vi "Post.vi"(8 "error in (no error)":errorcluster, 9 "PostRequest":string, 10 "Request":string, 11 "ByteGSWebAPI-V0 in":refnum<class "ByteGSWebAPI-V0.lvclass">) -> (0 "error out":errorcluster, 3 "ByteGSWebAPI-V0 out":refnum<class "ByteGSWebAPI-V0.lvclass">, 4 "body":string, 6 "headers":string)   [LabVIEW 2019, in "ByteGSWebAPI.lvlib" / "ByteGSWebAPI-V0.lvclass"]
uses:
  ByteGSWebAPI-V0.lvclass
  <vilib>/httpClient/POSTBuffer.vi
  <vilib>/httpClient/LabVIEWHTTPClient.lvlib
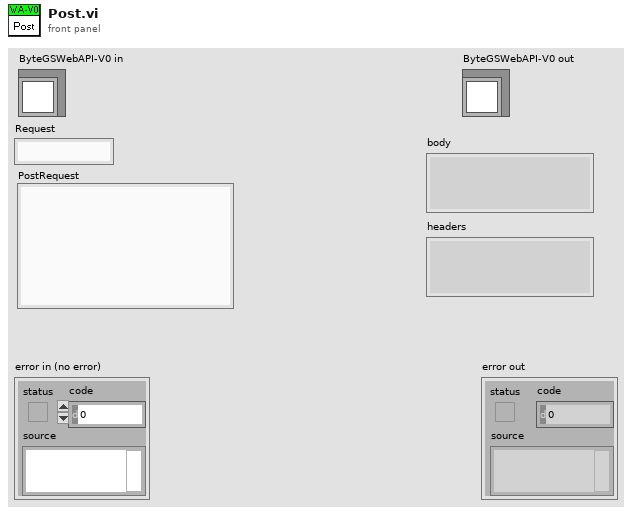
[diagram p1: front panel]
types:
  T1 = typedef "LabVIEWHTTPClient.lvlib/ClientHandle.ctl" = refnum<k1>
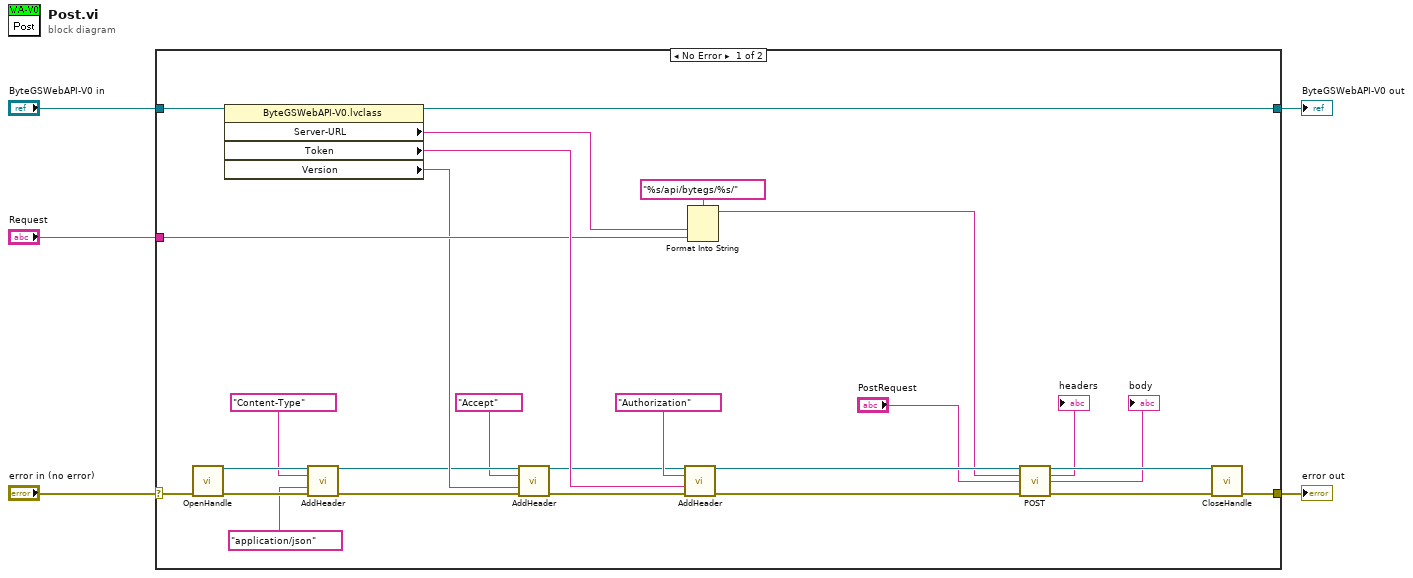
[diagram p0: block diagram]
diagram:
  n1 = case shown="No Error" "error in (no error)" {
    selector: "error in (no error)" -> [w27 w34]
    tunnel: [w26 w34] -> w4
    tunnel: [w25 w33] -> w2
    tunnel: "ByteGSWebAPI-V0 in" -> [w24 w33]
    tunnel: "Request" -> [w20 _]
    frame No Error {
      n2 = call <vilib>:"OpenHandle.vi"("error in (no error)"=w27) -> ("client handle out"=w30:T1, "error out"=w31:errorcluster)  [unwired: 13 in]
      n3 = property class="ByteGSWebAPI-V0.lvclass"(reference=w24) -> (reference out=w25:refnum<class "ByteGSWebAPI-V0.lvclass">, "Server-URL"=w21:string, "Token"=w23:string, "Version"=w19:string)  [unwired: 1 in, 1 out]
      n4 = call <vilib>:"AddHeader.vi"("client handle"=w30, "header"="Content-Type", "value"="application/json", "error in (no error)"=w31) -> ("client handle out"=w18:T1, "error out"=w17:errorcluster)  [unwired: 10 in]
      n5 = call <vilib>:"AddHeader.vi"("client handle"=w18, "header"="Accept", "value"=w19, "error in (no error)"=w17) -> ("client handle out"=w15:T1, "error out"=w16:errorcluster)  [unwired: 10 in]
      n6 = call <vilib>:"AddHeader.vi"("client handle"=w15, "header"="Authorization", "value"=w23, "error in (no error)"=w16) -> ("client handle out"=w13:T1, "error out"=w7:errorcluster)  [unwired: 10 in]
      n7 = Format Into String(format string="%s/api/bytegs/%s/" ("url"), w21, w20) -> (resulting string=w10:string)  [unwired: 2 in, 1 out]
      n8 = call-poly <vilib>:"POST.vi"("client handle"=w13, "url"=w10, "buffer"="PostRequest", "error in (no error)"=w7) -> ("client handle out"=w12:T1, "headers"=→"headers":string, "body"=→"body":string, "error out"=w11:errorcluster)  [unwired: 8 in]
      n9 = call <vilib>:"CloseHandle.vi"("client handle"=w12, "error in (no error)"=w11) -> ("error out"=w26:errorcluster)  [unwired: 13 in]
    }
    frame Error {
    }
  }
  "error out" <- w4
  "ByteGSWebAPI-V0 out" <- w2
